vi "子VI-线性灰度值曲线查看.vi"(9 "Palette:User Palette":cluster{"Red":u8, "Green":u8, "Blue":u8}[](array[cluster]), 10 "图像分辨率":T1, 11 "Image":T2(plugin-control)) -> ()   [LabVIEW 2021]
uses:
  <vilib>/vision/NI_Vision_Development_Module.lvlib
panel:
  out "游标间长度（mm）":dbl format="%#.2g"
  out "游标1":cluster{"X坐标":dbl, "Y坐标":dbl}
  out "游标0":cluster{"X坐标":dbl, "Y坐标":dbl}
  in  "退出":bool
  out "平均灰度值":sgl
  out "最大灰度值":sgl
  out "最小灰度值":sgl
  out "线性灰度值曲线":cluster{"x0":sgl, "dx":sgl, "Pixels Line":sgl[]}(graph)
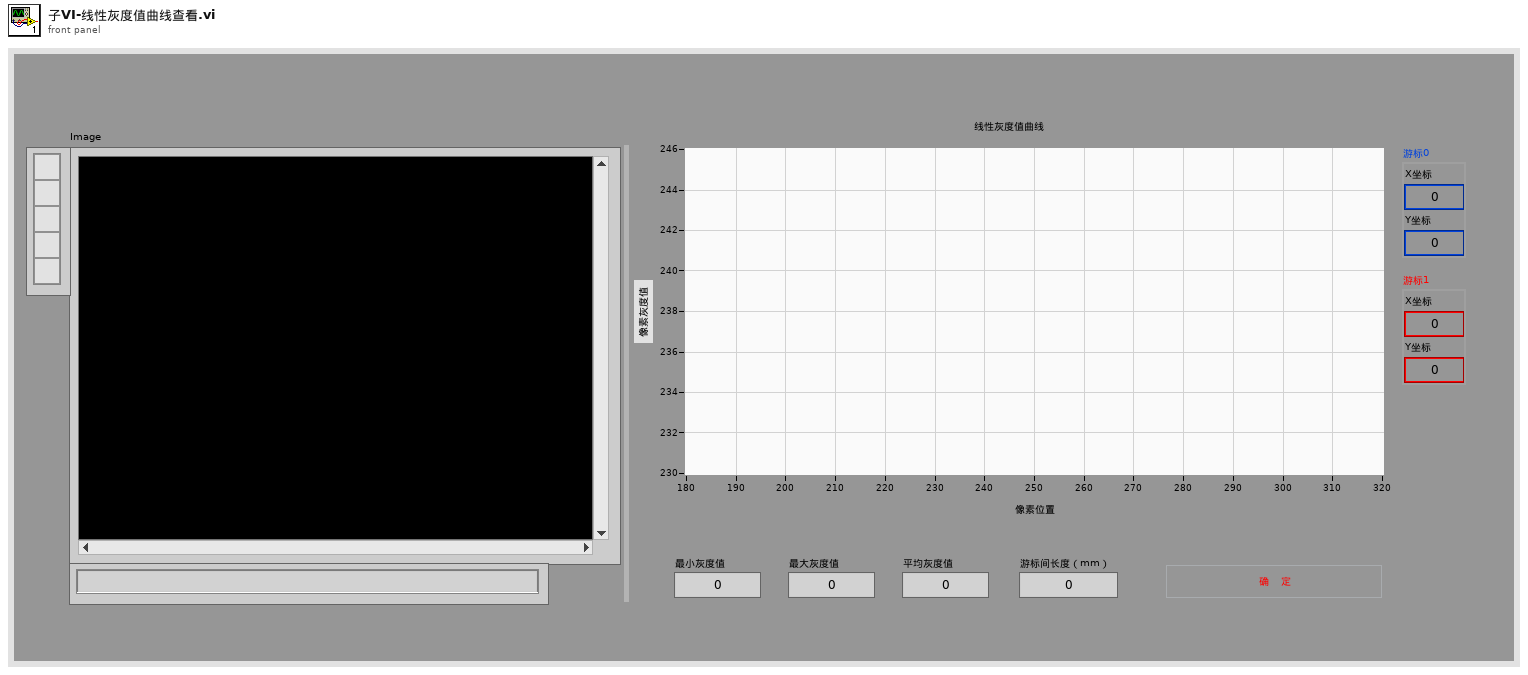
[diagram p1: front panel]
types:
  T1 = cluster{"图像X向分辨率（mm/像素）":dbl, "图像Y向分辨率（mm/像素）":dbl}
  T2 = typedef "IMAQ Image.ctl" = refnum<image>
  T3 = cluster{"Zoom Tool":bool, "Selection Tool":bool, "Pan Tool":bool, "Point Tool":bool, "Line Tool":bool, "Rectangle Tool":bool, "Rotated Rectangle Tool":bool, "Polyline Tool":bool, "Polygon Tool":bool, "Freehand Tool":bool, "Closed Freehand Tool":bool, "Ellipse Tool":bool, "Annulus Tool":bool}
  T4 = cluster{"Global Rectangle":i32[], "Contours":cluster{"Contour Type":u32, "ROI Type":u32, "Points":i32[]}[]}
  T5 = cluster{"x1Left":i32, "y1Top":i32, "x2Right":i32, "y2Bottom":i32}
  T6 = cluster{"Min":sgl, "Max":sgl, "Mean":sgl, "Std Dev":sgl, "Count":i32}
  T7 = typedef "LVCursorListTypeDef.ctl" = cluster{"Name":string, "Color":u32, "Style":u8, "Point Style":u8, "Name Visible":bool, "Allow Drag":bool, "Cursor Mode":u32, "Plot":i32, "Index":i32, "Position":cluster{"X":dbl, "Y":dbl}, "X Scale":u32, "Y Scale":u32, "Watch Plots":i32[], "Watch All Plots":bool, "Plot Area":i32, "Label Offset":cluster{"X":dbl, "Y":dbl}}[]
  T8 = cluster{"Name":string, "Color":u32, "Style":u8, "Point Style":u8, "Name Visible":bool, "Allow Drag":bool, "Cursor Mode":u32, "Plot":i32, "Index":i32, "Position":cluster{"X":dbl, "Y":dbl}, "X Scale":u32, "Y Scale":u32, "Watch Plots":i32[], "Watch All Plots":bool, "Plot Area":i32, "Label Offset":cluster{"X":dbl, "Y":dbl}}
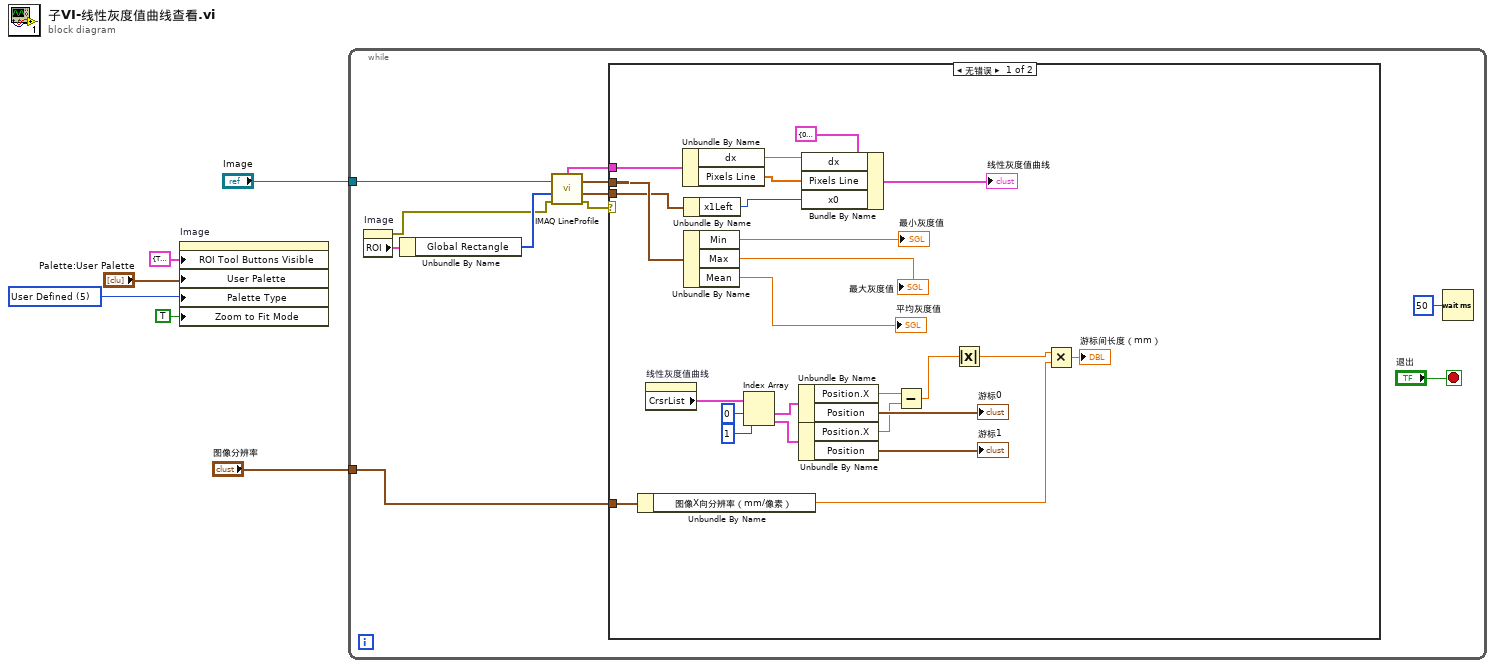
[diagram p0: block diagram]
diagram:
  w2 = u32 5 items=["Grayscale", "Binary", "Gradient", "Rainbow", "Temperature", "User Defined", "Binary 16 Bit", "Gradient 16 Bit", "Rainbow 16 Bit", "Temperature 16 Bit", "User Defined 16 Bit"] ("Palette:Palette Type")
  n1 = property on="Image" class="ImageControl"("ROI Tool Buttons Visible"=T3 {"Zoom Tool"=TRUE, "Selection Tool"=TRUE, "Pan Tool"=TRUE, "Point Tool"=FALSE, "Line Tool"=TRUE, "Rectangle Tool"=TRUE, "Rotated Rectangle Tool"=FALSE, "Polyline Tool"=FALSE, "Polygon Tool"=FALSE, "Freehand Tool"=FALSE, "Closed Freehand Tool"=FALSE, "Ellipse Tool"=FALSE, "Annulus Tool"=FALSE} ("ROI Tool Buttons Visible:All Elements"), "User Palette"="Palette:User Palette", "Palette Type"=w2, "Zoom to Fit Mode"=TRUE) -> ()  [unwired: 2 in, 2 out]
  n2 = while {
    tunnel: "Image" -> [w15]
    tunnel: "图像分辨率" -> [w7]
    stop <- "退出" stop-if-true
    n3 = property on="Image" class="ImageControl"() -> (error out=w11:errorcluster, "ROI"=w14:T4)  [unwired: 2 in, 1 out]
    n4 = Unbundle By Name(w14) -> ("Global Rectangle"=w13:i32[])
    n5 = call "IMAQ LineProfile"("error in (no error)"=w11, "Line Coordinates"=w13, "Image"=w15) -> ("Global Rectangle"=w8:T5, "error out"=w12:errorcluster, "Line Graph"=w9:cluster{"x0":sgl, "dx":sgl, "Pixels Line":sgl[]}, "Line Information"=w10:T6)  [unwired: 2 in]
    n6 = case shown="无错误" w12 {
      tunnel: w10 -> [w26 _]
      tunnel: w9 -> [w27 _]
      tunnel: w8 -> [w25 _]
      tunnel: w7 -> [w21 _]
      frame No Error {
        n7 = Unbundle By Name(w21) -> ("图像X向分辨率（mm/像素）"=w18:dbl)
        n8 = property on="线性灰度值曲线" class="WFGraph (严格)"() -> ("CrsrList"=w42:T7)  [unwired: 2 in, 2 out]
        n9 = Unbundle By Name(w27) -> ("dx"=w29:sgl, "Pixels Line"=w30:sgl[])
        n10 = Unbundle By Name(w25) -> ("x1Left"=w31:i32)
        n11 = Unbundle By Name(w26) -> ("Min"=→"最小灰度值":sgl, "Max"=→"最大灰度值":sgl, "Mean"=→"平均灰度值":sgl)
        n12 = Index Array(array=w42, index #1=0 ("索引"), index #2=1 ("索引")) -> (element #1=w39:T8, element #2=w38:T8)
        n13 = Unbundle By Name(w39) -> ("Position.X"=w24:dbl, "Position"=→"游标0":cluster{"X":dbl, "Y":dbl})
        n14 = Unbundle By Name(w38) -> ("Position.X"=w23:dbl, "Position"=→"游标1":cluster{"X":dbl, "Y":dbl})
        n15 = Bundle By Name(cluster=cluster{"x0":sgl, "dx":sgl, "Pixels Line":sgl[]} {"x0"=0.0, "dx"=0.0, "Pixels Line"=[]} ("Line Graph"), "dx"=w29, "Pixels Line"=w30, "x0"=w31) -> (→"线性灰度值曲线":cluster{"x0":sgl, "dx":sgl, "Pixels Line":sgl[]})
        n16 = Subtract(x=w24, y=w23) -> (x-y=w22:dbl)
        n17 = Absolute Value(x=w22) -> (abs(x)=w19:dbl)
        n18 = Multiply(x=w19, y=w18) -> (x*y=→"游标间长度（mm）":dbl)
      }
      frame Error {
      }
    }
    n19 = Wait (ms)(milliseconds to wait=u32 50 ("等待时间（毫秒）")) -> ()  [unwired: 1 out]
  }
